vi "PV Error Reset.vi"(7 "Adress of unit":u16=1 max=999 step=1, 8 "error in (no error)":errorcluster, 11 "VISA session":refnum<visa-resource-name>) -> (0 "error out":errorcluster, 3 "VISA resource out":refnum<visa-resource-name>)   [LabVIEW 2023, in "Pfeiffer Vacuum.lvlib"]
doc: "Resets the Error (Para 009 - error acknowledgement (write only))."
uses:
  <instrlib>/Pfeiffer Vacuum/Pfeiffer Vacuum.lvlib
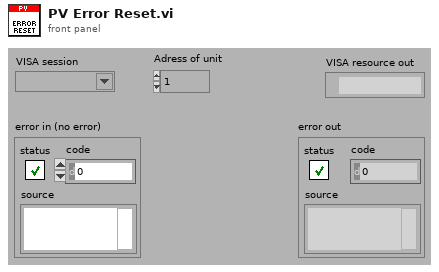
[diagram p1: front panel]
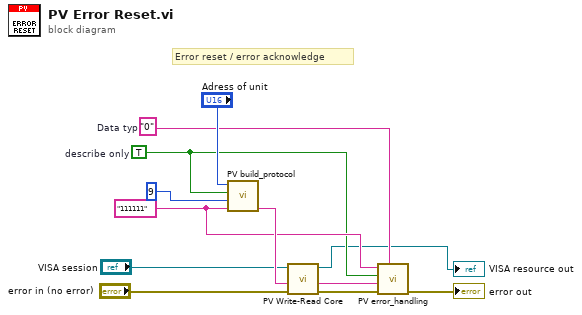
[diagram p0: block diagram]
diagram:
  w7 = "0"  # Data typ
  w6 = "111111" ("Data")
  w5 = TRUE  # describe only
  # "Error reset / error acknowledge"
  n1 = call <instrlib>:"PV build_protocol.vi"("Data"=w6, "Parameter-number"=u16 9, "parameter\nread<->describe"=w5, "Adress"="Adress of unit") -> ("output"=w10:string)  [unwired: 3 in]
  n2 = call <instrlib>:"PV Write-Read Core.vi"("error in"="error in (no error)", "Write data in"=w10, "VISA session"="VISA session") -> ("error out"=w8:errorcluster, "response (data) out"=w9:string, "dup VISA session"=→"VISA resource out":refnum<visa-resource-name>)  [unwired: 2 in]
  n3 = call <instrlib>:"PV error_handling.vi"("Data Typ in"=w7, "error in"=w8, "response (data) in"=w9, "Parameter\nread only<->describe"=w5, "data in"=w6) -> ("error out"=→"error out":errorcluster)  [unwired: 4 in, 2 out]
